vi "inteference -- find center.vi"(7 "number of points":i32, 8 "complex region":T1={"max re"=5.161869466666667e-06, "min re"=5.176843333333334e-06, "max im"=-2.467216e-05, "min im"=-0.001573233, "delta re"=0.003211203, "delta im"=0.00165815, "center re"=0.0015485608400000002, "delta  z"=0.0015530530000000002+0.0i, "center im"=0.0, "center z"=0.0+0.0i, "d im"=0.0, "d re"=0.0, "d z"=0.0+0.0i}, 9 "pond":cdb[][](array[numeric]), 10 "point sources":cdb[](array[numeric]), 11 "wave packet":cdb[][](array[numeric])) -> (2 "z (center)":cdb)   [LabVIEW 2010]
uses:
  complex region.ctl
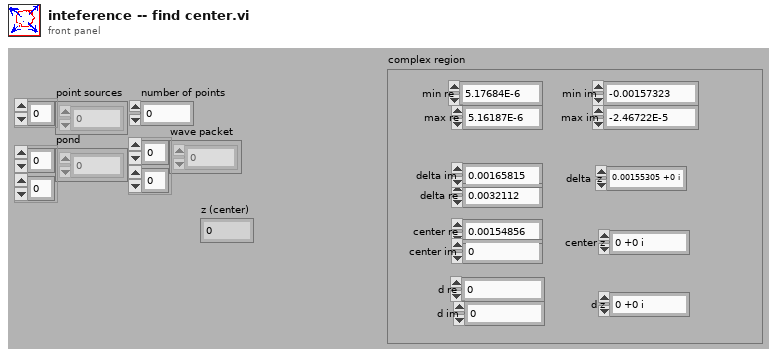
[diagram p1: front panel]
types:
  T1 = typedef "complex region.ctl" = cluster{"max re":dbl, "min re":dbl, "max im":dbl, "min im":dbl, "delta re":dbl, "delta im":dbl, "center re":dbl, "delta  z":cdb, "center im":dbl, "center z":cdb, "d im":dbl, "d re":dbl, "d z":cdb}
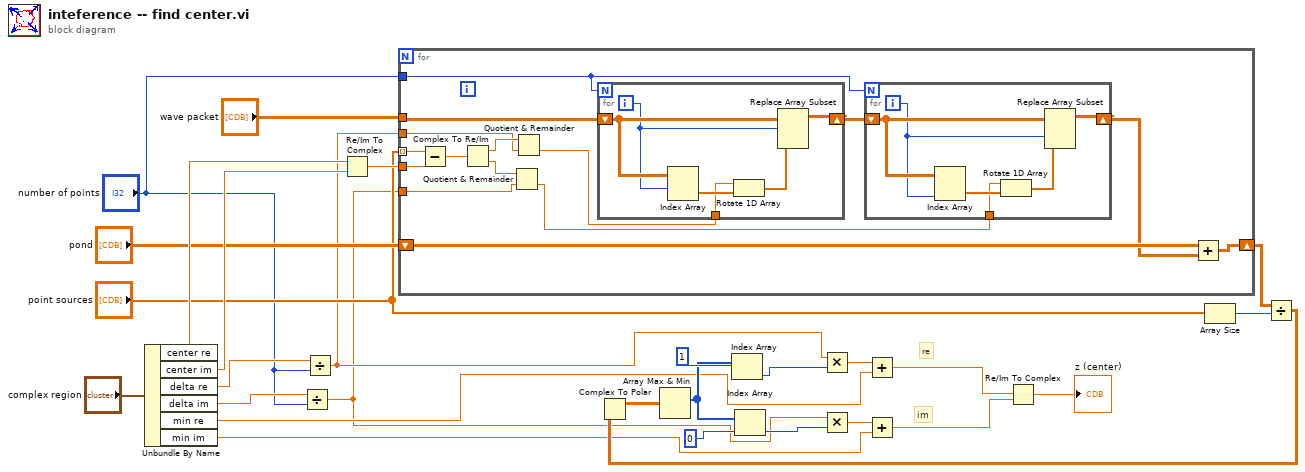
[diagram p0: block diagram]
diagram:
  # "re"
  # "im"
  n1 = Unbundle By Name("complex region") -> ("center re"=w28:dbl, "center im"=w27:dbl, "delta re"=w19:dbl, "delta im"=w18:dbl, "min re"=w4:dbl, "min im"=w3:dbl)
  n2 = Divide(x=w18, y="number of points") -> (x/y=w1:dbl)
  n3 = Divide(x=w19, y="number of points") -> (x/y=w2:dbl)
  n4 = Re/Im To Complex(1:w27, 2:w28) -> (0:w26:cdb)
  n5 = for {
    shift-right: [w42] -> w25
    shift-left: "pond" -> [w43]
    tunnel: "point sources" -> [w41] mode=indexing
    tunnel: "wave packet" -> [w31]
    tunnel: w26 -> [w40]
    tunnel: w2 -> [w37]
    tunnel: w1 -> [w35]
    tunnel: "number of points" -> [w33]
    n6 = Subtract(x=w41, y=w40) -> (x-y=w39:cdb)
    n7 = Complex To Re/Im(x + iy=w39) -> (x=w38:dbl, y=w36:dbl)
    n8 = Quotient & Remainder(x=w36, y=w35) -> (floor(x/y)=w29:dbl)  [unwired: 1 out]
    n9 = Quotient & Remainder(x=w38, y=w37) -> (floor(x/y)=w30:dbl)  [unwired: 1 out]
    n10 = for {
      N: w33 -> [_]
      shift-right: [w55] -> w34
      shift-left: w31 -> [w54]
      tunnel: w30 -> [w51]
      i -> [w50]
      n11 = Index Array(array=w54, index (row)=w50) -> (element=w52:cdb[])  [unwired: 1 in]
      n12 = Rotate 1D Array(1:w52, 2:w51) -> (0:w53:cdb[])
      n13 = Replace Array Subset(array=w54, new element=w53, index (row)=w50) -> (w55:cdb[][])  [unwired: 1 in]
    }
    n14 = for {
      N: w33 -> [_]
      shift-right: [w49] -> w32
      shift-left: w34 -> [w48]
      tunnel: w29 -> [w45]
      i -> [w44]
      n15 = Index Array(array=w48, index (col)=w44) -> (element=w46:cdb[])  [unwired: 1 in]
      n16 = Rotate 1D Array(1:w46, 2:w45) -> (0:w47:cdb[])
      n17 = Replace Array Subset(array=w48, new element=w47, index (col)=w44) -> (w49:cdb[][])  [unwired: 1 in]
    }
    n18 = Add(x=w43, y=w32) -> (x+y=w42:cdb[][])
  }
  n19 = Array Size(array="point sources") -> (size(s)=w24:i32)
  n20 = Divide(x=w25, y=w24) -> (x/y=w14:cdb[][])
  n21 = Complex To Polar(r * e^(i*theta)=w14) -> (r=w13:dbl[][])  [unwired: 1 out]
  n22 = Array Max & Min(array=w13) -> (max index (indices)=w12:i32[])  [unwired: 3 out]
  n23 = Index Array(array=w12, index=1) -> (element=w6:i32)
  n24 = Index Array(array=w12, index=0) -> (element=w5:i32)
  n25 = Multiply(x=w2, y=w6) -> (x*y=w11:dbl)
  n26 = Multiply(x=w1, y=w5) -> (x*y=w10:dbl)
  n27 = Add(x=w11, y=w4) -> (x+y=w9:dbl)
  n28 = Add(x=w10, y=w3) -> (x+y=w8:dbl)
  n29 = Re/Im To Complex(1:w8, 2:w9) -> (0:→"z (center)":cdb)
